vi "ALTS-2015 Auto Mode.vi"() -> ()   [LabVIEW 2013]
doc: "Copyright © 2005, Soliton Technologies.\nAll rights reserved."
uses:
  Controls/ALTS-2015 Station Details.ctl
  Controls/ALTS-2015 Status Ring Indicator.ctl
  Controls/ALTS-2015 Robot Actions.ctl
  SLL DAQ Engine/Software/Source Code/Sub VIs/DAQ Engine/Controls/SLL DE List of Digital Inputs.ctl
  Controls/ALTS-2015 Auto Main Screen States.ctl
  Sub VIs/OPC Engine/Controls/ALTS-2015 OPC Global Elements.ctl
  Sub VIs/OPC Engine/Controls/ALTS-2015 OPC Global Options.ctl
  Controls/ALTS-2015 Data Cluster.ctl
  Controls/ALTS-2015 Station Cluster.ctl
  Controls/ALTS-2015 INI Configuration Cluster.ctl
  Controls/ALTS-2015 Unload Task Data.ctl
  Controls/ALTS-2015 Status Message Options.ctl
  Controls/ALTS-2015 LV2GBL WorkOrder&SN Info Options.ctl
  Controls/ALTS-2015 LV2GBL Options.ctl
  Controls/ALTS-2015 WorkOrder&SN Cluster.ctl
  Controls/ALTS-2015 Control Reference LV2 Options.ctl
  Controls/ALTS-2015 Control Reference.ctl
  SLL DAQ Engine/Software/Source Code/Sub VIs/DAQ Engine/Controls/SLL DE DI Global Options.ctl
  Controls/ALTS-2015 LV2GBL Restart Options.ctl
  Controls/ALTS-2015 LV2 Options.ctl
  <vilib>/Utility/error.llb/DialogType.ctl
  SLL DAQ Engine/Software/Source Code/Sub VIs/DAQ Engine/Controls/SLL DE DO Global Options.ctl
  Controls/ALTS-2015 Auto Program States.ctl
  Sub VIs/Robot Controller Queue/ALTS-2015 Robot Cotroller Options.ctl
  SLL DAQ Engine/Software/Source Code/Sub VIs/DAQ Engine/Controls/SLL DE DAQ Global Options.ctl
  SLL DAQ Engine/Software/Source Code/Sub VIs/DAQ Engine/Controls/SLL DE DAQ Global Elements.ctl
  Controls/ALTS-2015 DO Start Stop Options.ctl
  Controls/ALTS-2015 LV2GBL Station Info Options.ctl
  Controls/ALTS-2015 Ring Indicator Enum.ctl
  Controls/ALTS-2015 Digital Output Options.ctl
  Controls/ALTS-2015 DB Driver Options.ctl
  Controls/ALTS-2015 Robot Tasks.ctl
  Controls/ALTS-2015 Serial Details.ctl
  Controls/ALTS-2015 Serial DB Details.ctl
  Controls/ALTS-2015 Serial Task Handler FGV-Command.ctl
  Controls/ALTS-2015 Write DB Write Result Driver Cases.ctl
  Controls/ALTS-2015 Bundle Cluster for DB Result Options.ctl
  Controls/ALTS-2015 write DB Result cases.ctl
  Globals/ALTS-2015 Global Variables.vi
  Sub VIs/OPC Engine/Globals/ALTS-2015 OPC Engine Globals.vi
panel:
  in  "Error Message":string
  out "User :":string caption="Date :"
  in  "Login/Logoff":bool
  in  "Restart":bool
  out "Status":string
  out "Error Occured":bool
  in  "Open Manual Screen":bool
  in  "List of Digital Inputs":T1
  out "Time :":string
  out "Date :":string
  in  "DI Status":bool[](array[boolean])
  out "Last Scanned Serial Number":string caption="Status"
  out "Station Cluster 4":T2={"Station Number"="", "Work Order Number"="", "Sensor Name"="", "Pressure (PSI)"="", "Flow (SCCM)"="", "Test Time "="", "Test Result"="", "Serial Number"="", "Station Status"=0, "SW assigned UUT"=FALSE, "Rerun Count"=0, "Test Type"=0, "Load Decision"=0, "Robot Action"=enum."No Action"}
  out "Station Cluster 3":T2={"Station Number"="", "Work Order Number"="", "Sensor Name"="", "Pressure (PSI)"="", "Flow (SCCM)"="", "Test Time "="", "Test Result"="", "Serial Number"="", "Station Status"=0, "SW assigned UUT"=FALSE, "Rerun Count"=0, "Test Type"=0, "Load Decision"=0, "Robot Action"=enum."No Action"}
  out "Station Cluster 2":T2={"Station Number"="", "Work Order Number"="", "Sensor Name"="", "Pressure (PSI)"="", "Flow (SCCM)"="", "Test Time "="", "Test Result"="", "Serial Number"="", "Station Status"=0, "SW assigned UUT"=FALSE, "Rerun Count"=0, "Test Type"=0, "Load Decision"=0, "Robot Action"=enum."No Action"}
  out "Station Cluster 1":T2={"Station Number"="", "Work Order Number"="", "Sensor Name"="", "Pressure (PSI)"="", "Flow (SCCM)"="", "Test Time "="", "Test Result"="", "Serial Number"="", "Station Status"=0, "SW assigned UUT"=FALSE, "Rerun Count"=0, "Test Type"=0, "Load Decision"=0, "Robot Action"=enum."No Action"}
  in  "Exit":bool
  out "error out":errorcluster
  in  "error in":errorcluster
  # "Air Leak Test System (Auto)"
  # "V 3.0.2"
  # "Dont delete these Controls. Its Property Nodes are used"
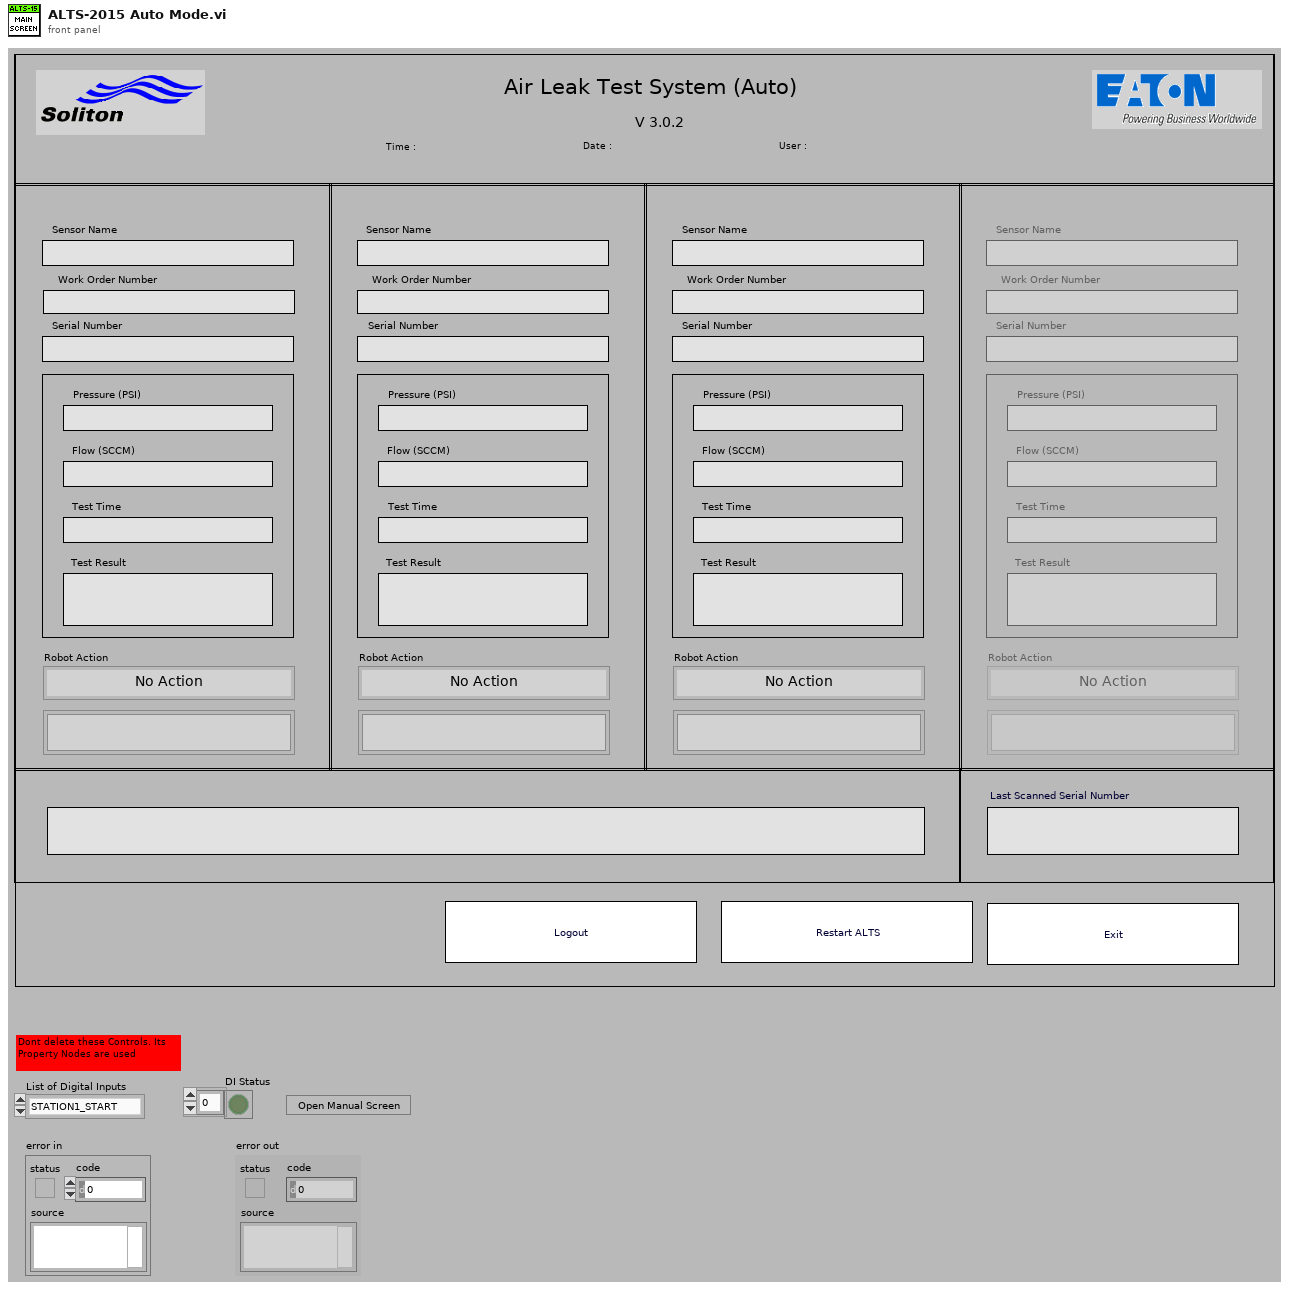
[diagram p1: front panel]
types:
  T1 = typedef "SLL DE List of Digital Inputs.ctl" = enum16{"STATION1_START", "STATION1_STOP", "STATION1_CLAMPED", "STATION1_TC_PASS", "STATION1_TC_FAIL", "STATION1_TTA", "STATION1_TTB", "STATION2_START", "STATION2_STOP", "STATION2_CLAMPED", "STATION2_TC_PASS", "STATION2_TC_FAIL", "STATION2_TTA", "STATION2_TTB", "STATION3_START", "STATION3_STOP", "STATION3_CLAMPED", "STATION3_TC_PASS", "STATION3_TC_FAIL", "STATION3_TTA", "STATION3_TTB", "STATION4_START", "STATION4_STOP", "STATION4_CLAMPED", "STATION4_TC_PASS", "STATION4_TC_FAIL", "STATION4_TTA", "STATION4_TTB"}
  T2 = typedef "ALTS-2015 Station Details.ctl" = cluster{"Station Number":string, "Work Order Number":string, "Sensor Name":string, "Pressure (PSI)":string, "Flow (SCCM)":string, "Test Time ":string, "Test Result":string, "Serial Number":string, "Station Status":T3, "SW assigned UUT":bool, "Rerun Count":i32, "Test Type":i32, "Load Decision":i32, "Robot Action":T4}
  T3 = typedef "ALTS-2015 Status Ring Indicator.ctl" = u16
  T4 = typedef "ALTS-2015 Robot Actions.ctl" = enum16{"Loading...", "Unloading...", "Reruning...", "No Action"}
  T5 = enum16{"Init", "Set - DB Loop", "Set - Robot Loop", "Get"}
  T6 = typedef "ALTS-2015 Auto Main Screen States.ctl" = enum16{">Initialize", ">Poll", ">Error", ">Exit", ">Restart", ">Authentication", ">Check Robot Requests", ">Scan Serial No", "<-------DI /OPC Actions------->", ">Check DI Status", ">Start the Test", ">Restore station after Stop", ">Stop the Test", ">UUT Clamped", ">UUT Unclamped", ">Read Test Data Result - Pass", ">Read Test Data Result - Fail", ">Update Rerun on Fail", ">Update Station Info", "<--------Enqueue Robot Task-------->", ">Enqueue New Serial Task", ">Enqueue Invalid Serial Task", ">Enqueue Rerun Task", ">Enqueu Unload Task"}
  T7 = enum16{"Init", "Set Task Pass", "Set Task Failure", "Set Task Status", "Get"}
  T8 = typedef "ALTS-2015 Control Reference.ctl" = cluster{"User :":refnum<vi>, "Station Cluster 1":refnum<vi>, "Station Cluster 2":refnum<vi>, "Station Cluster 3":refnum<vi>, "Station Cluster 4":refnum<vi>, "Error Message":refnum<vi>, "Login/Logoff":refnum<vi>}
  T9 = typedef "ALTS-2015 Control Reference LV2 Options.ctl" = enum16{"Set", "Get"}
  T10 = enum32{"invalid app kind", "Development System", "Run Time System", "Student Edition", "Embedded LabVIEW", "Evaluation", "Custom"}
  T11 = typedef "ALTS-2015 WorkOrder&SN Cluster.ctl" = cluster{"Work Order Number":string}
  T12 = typedef "ALTS-2015 LV2GBL Options.ctl" = enum16{"Read all", "Write all"}
  T13 = typedef "ALTS-2015 LV2GBL WorkOrder&SN Info Options.ctl" = enum16{"Init", "Read all", "Write Work Order"}
  T14 = typedef "ALTS-2015 Status Message Options.ctl" = enum16{"Initializing...", "Enter User Login...", "Valid Serial Number...", "Invalid Serial Number...", "Start Tag Received...", "Stop Tag Received...", "UUT Clamped...", "UUT not Clamped...", "Test Running...", "Test Complete...", "Task is assigned to robot...", "Robot is working on the task...", "Robot is ready for next task...", "Writing Result to DB...", "Idle...", "Exiting..."}
  T15 = typedef "SLL DE DI Global Options.ctl" = enum16{"Init", "Write Line", "Write Array", "Read Line", "Read Array", "Read Full Status", "Write Full Status"}
  T16 = typedef "ALTS-2015 LV2GBL Restart Options.ctl" = enum16{"Get All Data", "Set Restart Notifier Ref", "Store Authentication Data"}
  T17 = enum32{"Invalid", "Standard", "Closed", "Hidden", "Minimized", "Maximized"}
  T18 = typedef "ALTS-2015 LV2 Options.ctl" = enum16{"Get", "Set"}
  T19 = typedef "SLL DE DAQ Global Elements.ctl" = enum16{"AI Error", "AO Error", "DI Error", "DO Error", "AI Restart", "DI Restart", "AI Running", "AO Running", "DI Running", "DO Running", "DAQ Exit?"}
  T20 = typedef "SLL DE DAQ Global Options.ctl" = enum16{"Init", "Write 1", "Read 1", "Write Array", "Read Array", "Clear"}
  T21 = typedef "ALTS-2015 Robot Cotroller Options.ctl" = enum16{"Init", "Enqueue State", "Enqueue State in Opposite End", "Dequeue State", "Exit"}
  T22 = typedef "ALTS-2015 Auto Program States.ctl" = enum16{"<------ Robot Handler States ------>", "Wait for Robot Availability", "Check Last Task by Robot", "Wait & Read Task from Queue", "Write New Task Details to Robot", "Write Task Available for Robot", "Check Robot for Unavailbilty", "Write Task Unavailable for Robot", "<------------ Other ------------>", "Error", "Exit"}
  T23 = typedef "ALTS-2015 Station Cluster.ctl" = enum16{"Station 1", "Station 2", "Station 3", "Station 4"}
  T24 = cluster{"Test Status":string, "Station Name":T23}
  T25 = typedef "SLL DE DO Global Options.ctl" = enum16{"Init", "Write Line", "Write Array", "Write Full Status", "Read Line", "Read Array", "Read Full Status", "Restart DO", "Send to Safe Mode", "Stop DO"}
  T26 = typedef "ALTS-2015 DO Start Stop Options.ctl" = enum16{"Start Test", "Stop Test"}
  T27 = typedef "ALTS-2015 Digital Output Options.ctl" = enum16{"Idle", "Test Running", "Pass", "Fail"}
  T28 = typedef "ALTS-2015 Ring Indicator Enum.ctl" = enum16{"Idle", "Test Running", "Unit Clamped", "Unit not Clamped", "Pass", "Fail"}
  T29 = typedef "ALTS-2015 LV2GBL Station Info Options.ctl" = enum16{"Init", "Read", "Read All", "Write Sensor ID", "Write  Work Order", "Write Serial Number", "Write Test Data", "Write Station Status", "Write Station Occupancy", "Write Station Test Type", "Write Rerun", "Write Load Decision", "Write Robot Action", "Clear All", "Clear Test Result"}
  T30 = typedef "ALTS-2015 Unload Task Data.ctl" = cluster{"Station to Unload":T23, "Test Result":bool}
  T31 = typedef "ALTS-2015 Serial Task Handler FGV-Command.ctl" = enum16{"Set Replace/Insert Falg", "Get Status", "Reset Flag", "Reset S Data"}
  T32 = typedef "ALTS-2015 Robot Tasks.ctl" = enum16{"Load", "Unload", "Rerun", "Invalid Serial"}
  T33 = typedef "ALTS-2015 DB Driver Options.ctl" = enum16{"Init", "Read DB", "Close"}
  T34 = typedef "ALTS-2015 Data Cluster.ctl" = cluster{"Serial No":string, "DI Change Status":bool[], "Station Selected":T23[], "Station to Start Stop Test":T23, "INI Info":T35, "Stations to Rerun":T23[], "Unload Task":T30[], "Dev. System?":bool, "Manual Restart?":bool}
  T35 = typedef "ALTS-2015 INI Configuration Cluster.ctl" = cluster{"Application":cluster{"Rerun Count":i32, "Workorder No":string, "PLC Scanner":bool, "Time Delay to Restart(mins)":dbl}, "Station Details":cluster{"Sensor Name 1":string, "Sensor Name 2":string, "Sensor Name 3":string, "Sensor Name 4":string, "Station1 Enable":bool, "Station2 Enable":bool, "Station3 Enable":bool, "Station4 Enable":bool}, "Database":cluster{"Database Connection Link":path, "Result Procedure":string, "User":string, "Password":string, "Prompt":bool, "Station 1 LT Result DB DSN Path":path, "Station 2 LT Result DB DSN Path":path, "Station 3 LT Result DB DSN Path":path, "Station 4 LT Result DB DSN Path":path, "AirLeakTestResult Procedure":string, "Serial Details Procedure":string}, "Simulation":cluster{"Simulate DAQ Hardware":bool, "Simulate Result DB Write":bool, "Simulate Scanner":bool, "Simulate OPC":bool, "Simulate Serial Details DB":bool, "Simulate Result DB":bool, "Simulate Scanner DB Path":path, "Simulate Serial Details DB Path":path, "Simulate Result DB Path":path}, "Barcode Scanner1":cluster{"Scanner IP":string, "Scanner Port":u16, "#Bytes to Read":i32, "Timeout_ms":i32}, "Barcode Scanner2":cluster{"Enabled?":bool, "Scanner IP":string, "Scanner Port":u16, "#Bytes to Read":i32}}
  T36 = typedef "DialogType.ctl" = u16
  T37 = cluster{"Station Cluster":T23, "Last Test Result":bool}
  T38 = typedef "ALTS-2015 Serial Details.ctl" = cluster{"Robot Task":T32, "Serial No":string, "New Serial?":bool, "Station # Unload":T23, "Last Test Result":bool, "Rerun?":bool, "Station # Rerun":T23, "Invalid Serial?":bool, "Serial Details":T39}
  T39 = typedef "ALTS-2015 Serial DB Details.ctl" = cluster{"Adapter Plate Size":i32, "Air Leak Test Type ":i32, "Displacement Size":i32, "Flange Size":i32, "Height":i32, "Load Decision":i32, "Cart Insert":i32}
  T40 = typedef "ALTS-2015 OPC Global Elements.ctl" = enum16{"OPC - R Error", "OPC - W Error", "OPC - R Restart", "OPC - W Restart", "OPC - R Running", "OPC - W Running"}
  T41 = typedef "ALTS-2015 OPC Global Options.ctl" = enum16{"Init", "Write 1", "Read 1", "Write Array", "Read Array", "Clear"}
  T42 = typedef "ALTS-2015 write DB Result cases.ctl" = enum16{"Enter All Data", "Enter WO & SN"}
  T43 = typedef "ALTS-2015 Bundle Cluster for DB Result Options.ctl" = enum16{"Write", "Read"}
  T44 = typedef "ALTS-2015 Write DB Write Result Driver Cases.ctl" = enum16{"Init", "Write Result", "Close"}
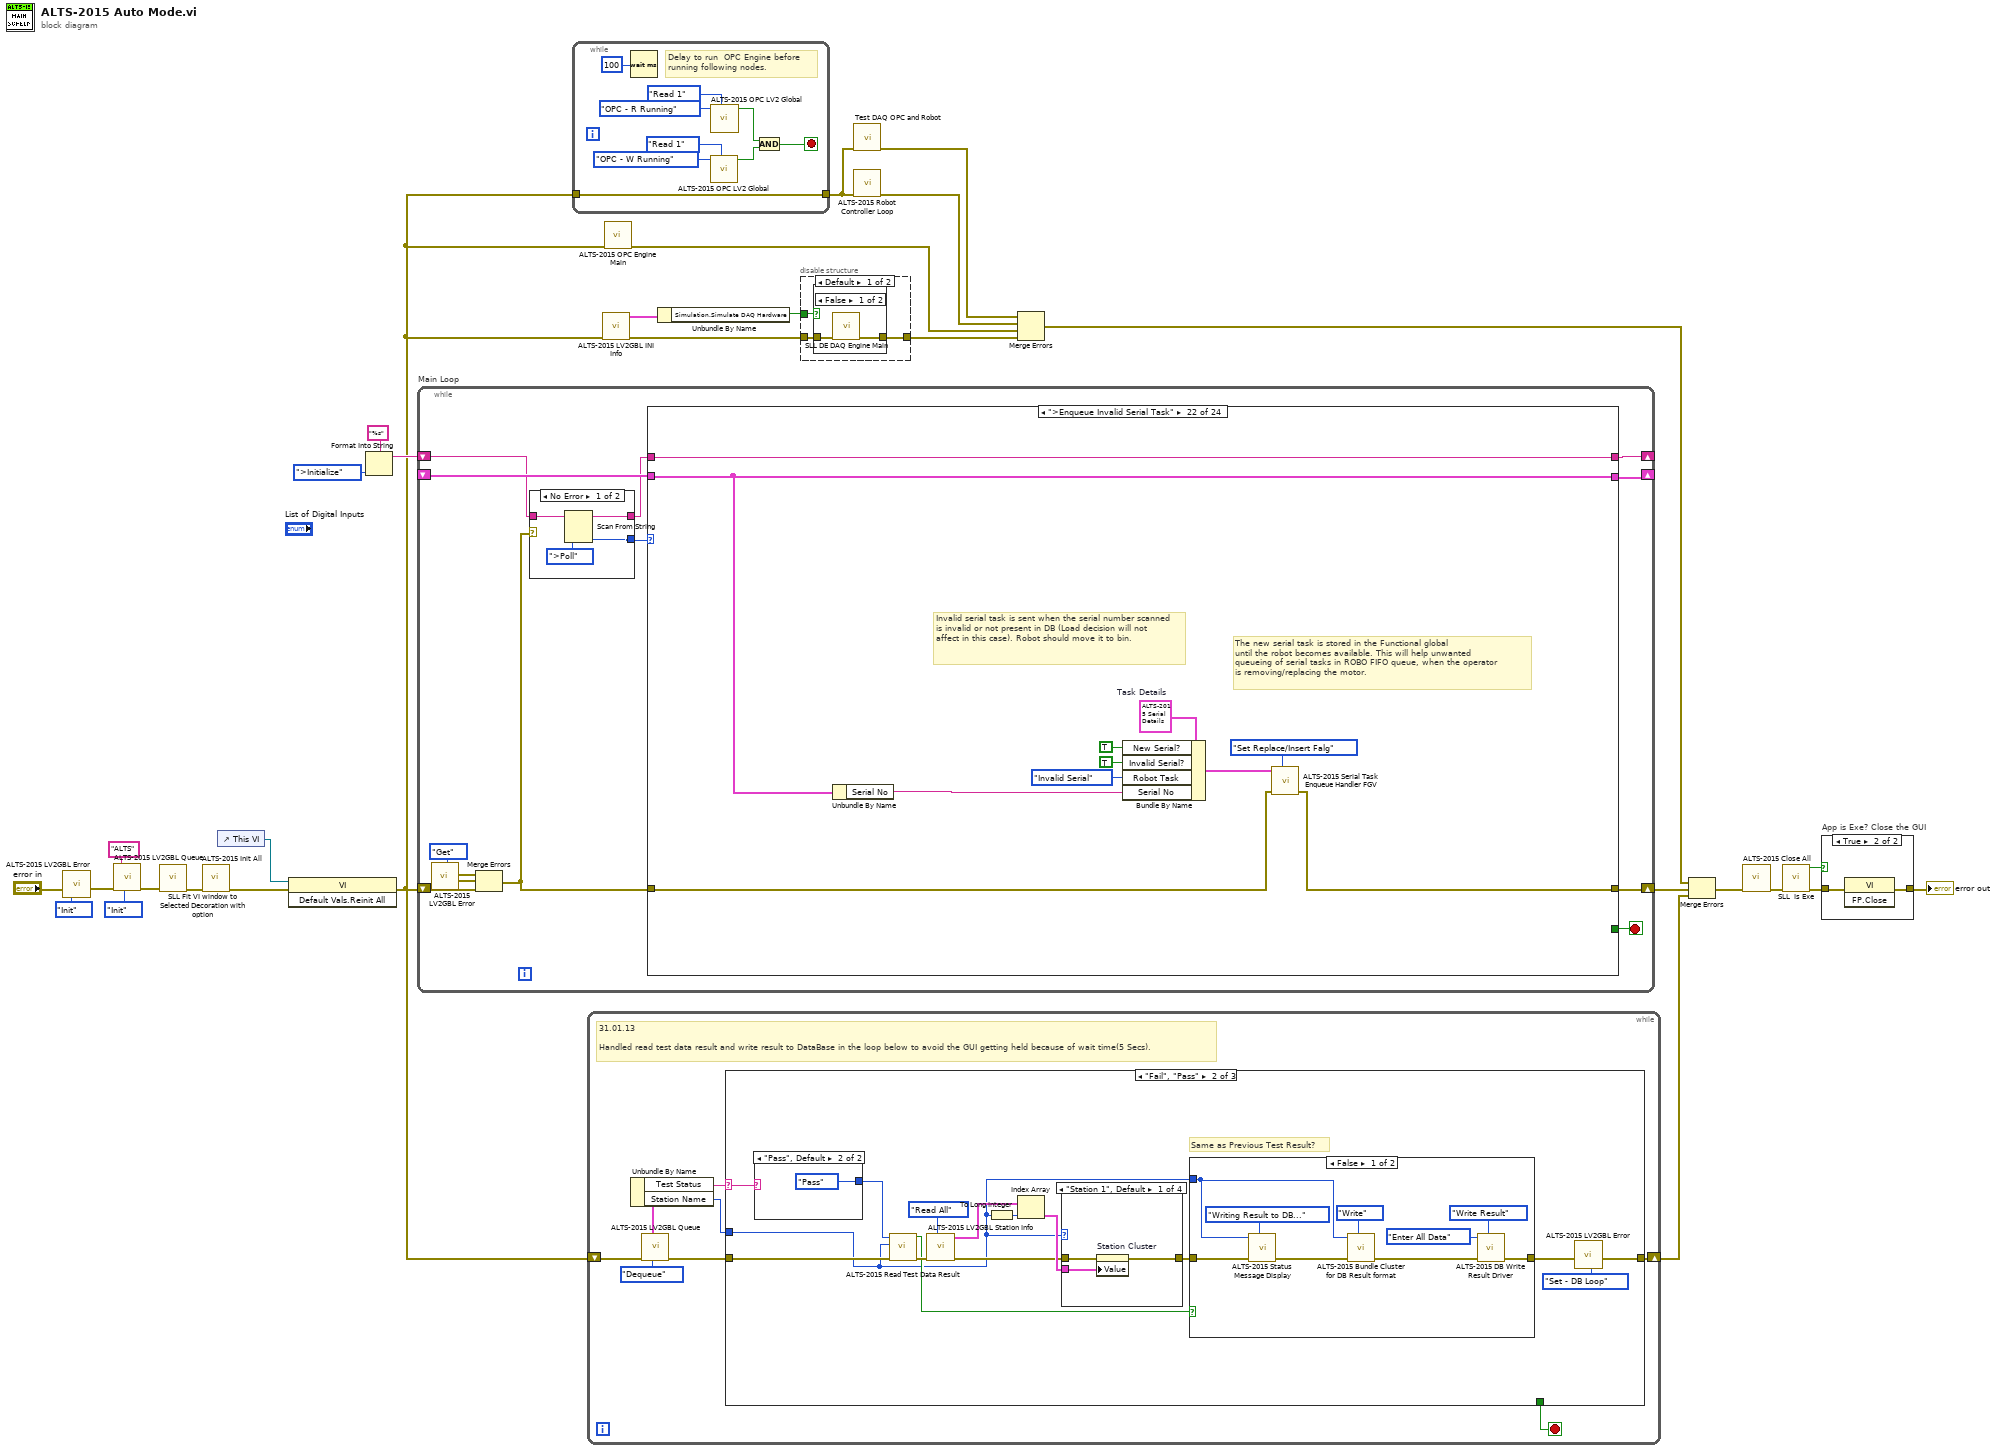
[diagram p0: block diagram]
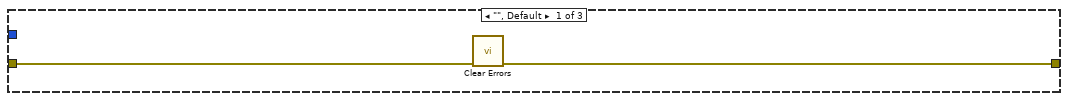
[diagram p5: hidden frame]
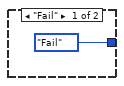
[diagram p6: hidden frame]
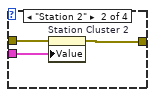
[diagram p8: hidden frame]
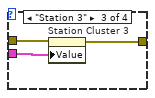
[diagram p9: hidden frame]
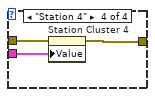
[diagram p10: hidden frame]
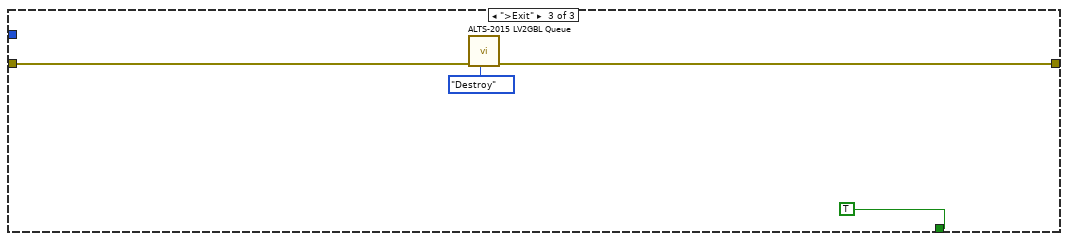
[diagram p11: hidden frame]
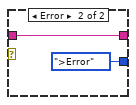
[diagram p12: hidden frame]
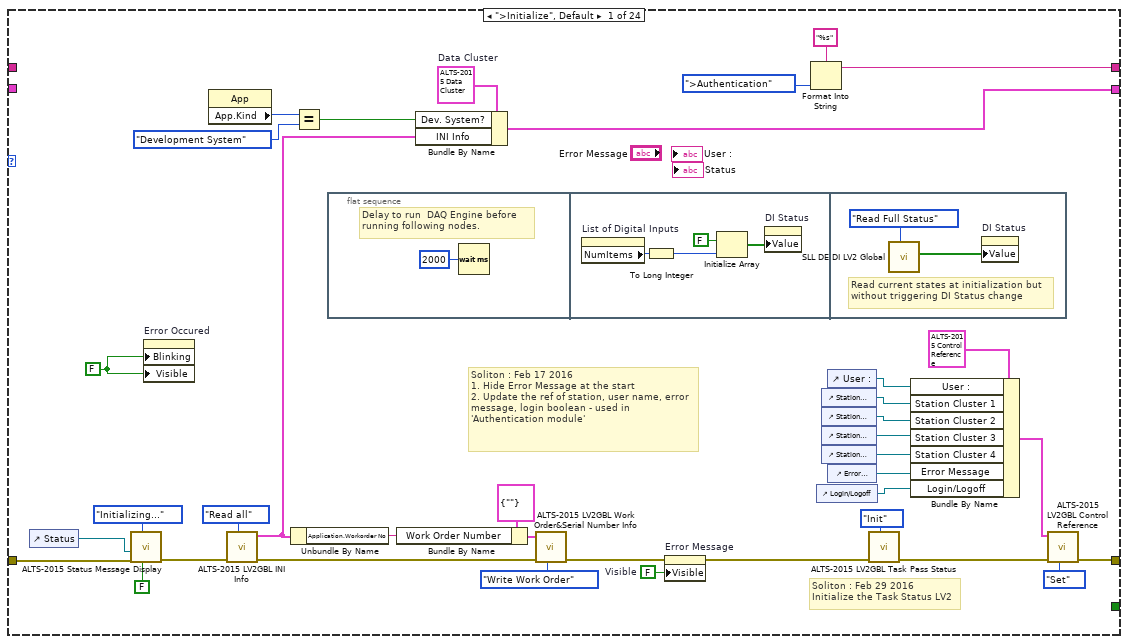
[diagram p13: hidden frame]
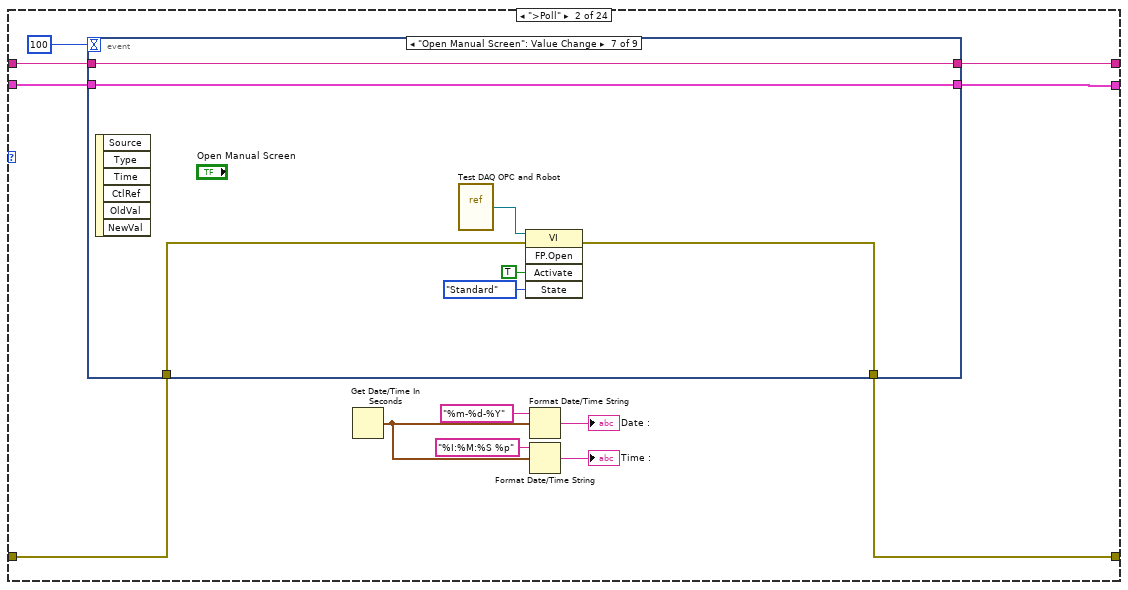
[diagram p14: hidden frame]
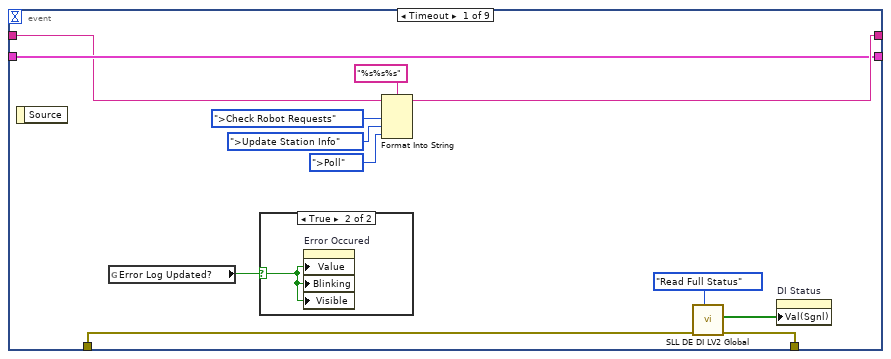
[diagram p15: hidden frame]
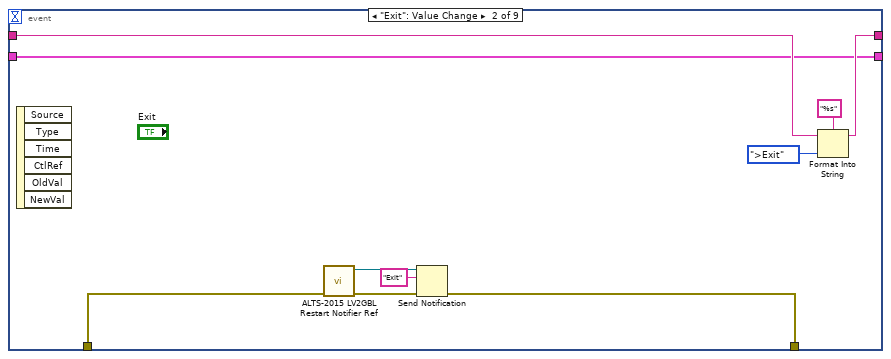
[diagram p17: hidden frame]
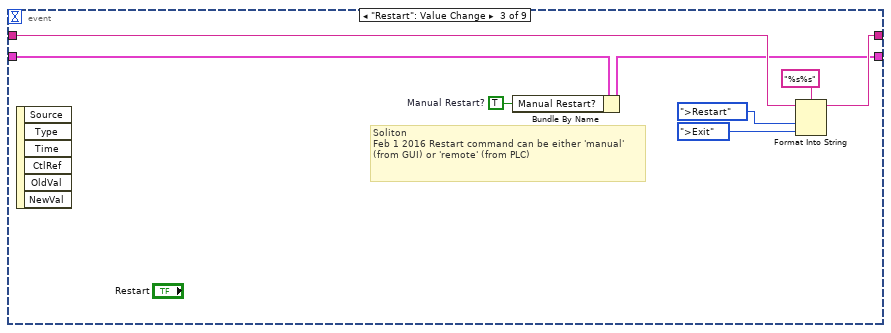
[diagram p18: hidden frame]
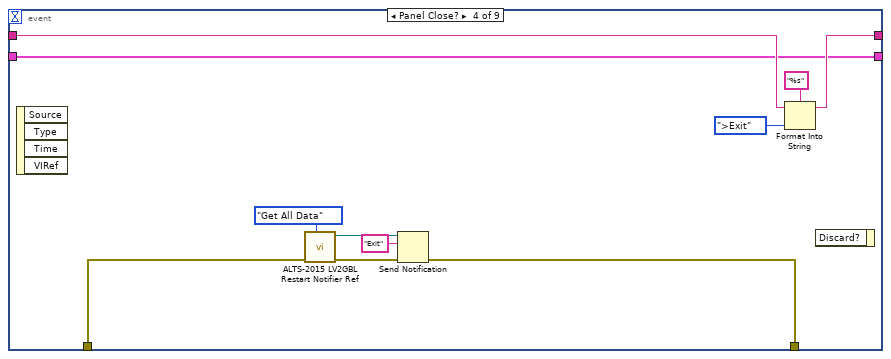
[diagram p19: hidden frame]
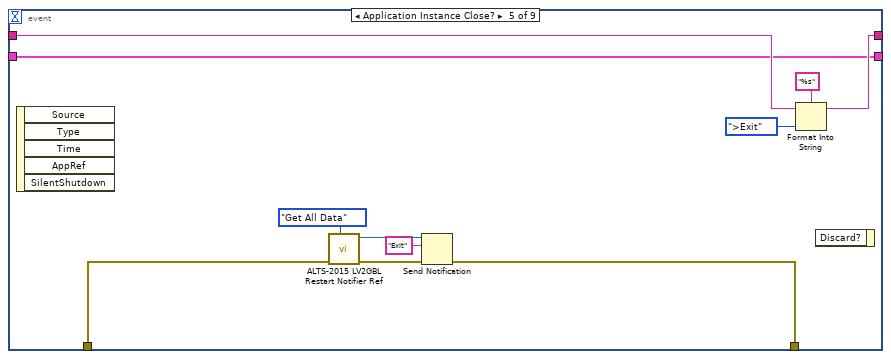
[diagram p20: hidden frame]
diagram:
  n1 = call "ALTS-2015 LV2GBL Error.vi"("error in - DB Loop"="error in", "Operation"=T5."Init") -> ("error out  - DB Loop"=w27:errorcluster)  [unwired: 8 in, 1 out]
  n2 = call "ALTS-2015 LV2GBL Queue.vi"("Enum"=enum16{"Init", "Enqueue", "Dequeue", "Destroy"}."Init", "error in (no error)"=w27, "Queue name"="ALTS") -> ("error out"=w23:errorcluster)  [unwired: 7 in, 1 out]
  n3 = call "SLL Fit VI window to Selected Decoration with option.vi"("error in (no error)"=w23) -> ("error out"=w22:errorcluster)  [unwired: 9 in, 1 out]
  n4 = call "ALTS-2015 Init All.vi"("error in"=w22) -> ("error out"=w13:errorcluster)  [unwired: 10 in]
  n5 = control-ref of="This VI"() -> (w4:refnum<vi>)
  n6 = invoke class="VI" method="Default Vals.Reinit All"(reference=w4, error in=w13) -> (error out=w5:errorcluster)  [unwired: 1 in, 2 out]
  n7 = Format Into String(format string="%s", ALTS-2015_Auto_Main_Screen_States.">Initialize") -> (resulting string=w17:string)  [unwired: 2 in, 1 out]
  n8 = while "Main Loop" {
    shift-right: [w42] -> _
    shift-left: w17 -> [w36]
    shift-right: [w40] -> w18
    shift-left: w5 -> [w31]
    shift-right: [w39] -> _
    shift-left: _ -> [w38]
    stop <- w37 stop-if-true
    n9 = call "ALTS-2015 LV2GBL Error.vi"("Operation"=T5."Get") -> ("error out  - DB Loop"=w32:errorcluster, "error out  - Robot Loop"=w34:errorcluster)  [unwired: 9 in]
    n10 = Merge Errors(w34, w32, w31) -> (w30:errorcluster)
    n11 = case shown="No Error" w30 {
      tunnel: [w45 ALTS-2015_Auto_Main_Screen_States.">Error"] -> w41
      tunnel: w36 -> [w44 w48]
      tunnel: [w43 w48] -> w35
      frame No Error {
        n12 = Scan From String(input string=w44, default 1=ALTS-2015_Auto_Main_Screen_States.">Poll") -> (remaining string=w43:string, output 1=w45:T6)  [unwired: 3 in, 2 out]
      }
      frame Error {
      }
    }
    n13 = case shown="\">Enqueue Invalid Serial Task\"" w41 {
      tunnel: [w81 w103 w239 w270 w283 w299 w305 w310 w318 w327 w349 w358 w389 w398 w410 w427 w446 w468 w501 w511 w518 w536 w537 w554] -> w42
      tunnel: w35 -> [_ w102 w239 w270 w283 w299 w305 w311 w312 w328 w349 w358 w389 w398 w410 w428 w446 w467 w501 w511 w518 w536 w538 w555]
      tunnel: [w64 w93 w230 w247 w281 w301 w304 w306 w314 w324 w348 w352 w367 w390 w405 w433 w447 w461 w497 w510 w522 w531 w544 w558] -> w40
      tunnel: w30 -> [w79 w104 w238 w249 w280 w300 w304 w307 w315 w323 w345 w354 w371 w391 w406 w421 w443 w462 w498 w510 w524 w535 w545 w560]
      tunnel: [w72 w99 w237 w269 w275 w302 w303 w308 w316 w321 w347 w350 w372 w392 w403 w431 w445 w458 w496 w509 w521 w528 w541 w556] -> w39
      tunnel: w38 -> [_ w100 w237 w269 w275 w302 w303 w309 w317 w322 w347 w351 w373 w393 w404 w432 w448 w460 w496 w509 w521 w528 w543 w559]
      tunnel: [_ _ _ TRUE ("Exit") _ _ _ _ _ _ _ _ _ _ _ _ _ _ _ _ _ _ _ _] -> w37
      frame ">Initialize", Default {
        w53 = FALSE  # Visible
        w65 = FALSE ("Blinking")
        w85 = T34 {"Serial No"="", "DI Change Status"=[], "Station Selected"=[], "Station to Start Stop Test"=enum."Station 1", "INI Info"={"Application"={"Rerun Count"=0, "Workorder No"="", "PLC Scanner"=FALSE, "Time Delay to Restart(mins)"=0.0}, "Station Details"={"Sensor Name 1"="", "Sensor Name 2"="", "Sensor Name 3"="", "Sensor Name 4"="", "Station1 Enable"=FALSE, "Station2 Enable"=FALSE, "Station3 Enable"=FALSE, "Station4 Enable"=FALSE}, "Database"={"Database Connection Link"=path "", "Result Procedure"="", "User"="", "Password"="", "Prompt"=FALSE, "Station 1 LT Result DB DSN Path"=path "", "Station 2 LT Result DB DSN Path"=path "", "Station 3 LT Result DB DSN Path"=path "", "Station 4 LT Result DB DSN Path"=path "", "AirLeakTestResult Procedure"="", "Serial Details Procedure"=""}, "Simulation"={"Simulate DAQ Hardware"=FALSE, "Simulate Result DB Write"=FALSE, "Simulate Scanner"=FALSE, "Simulate OPC"=FALSE, "Simulate Serial Details DB"=FALSE, "Simulate Result DB"=FALSE, "Simulate Scanner DB Path"=path "", "Simulate Serial Details DB Path"=path "", "Simulate Result DB Path"=path ""}, "Barcode Scanner1"={"Scanner IP"="", "Scanner Port"=0, "#Bytes to Read"=0, "Timeout_ms"=0}, "Barcode Scanner2"={"Enabled?"=FALSE, "Scanner IP"="", "Scanner Port"=0, "#Bytes to Read"=0}}, "Stations to Rerun"=[], "Unload Task"=[], "Dev. System?"=FALSE, "Manual Restart?"=FALSE}  # Data Cluster
        # "Soliton : Feb 29 2016\nInitialize the Task Status LV2"
        # "Soliton : Feb 17 2016\n1. Hide Error Message at the start\n2. Update the ref of station, user name, error message, login boolean - used in 'Authentication module'"
        n14 = control-ref of="Status"() -> (w69:refnum<vi>)
        n15 = call "ALTS-2015 Status Message Display.vi"("Station Message?"=FALSE, "Status Message Options"=ALTS-2015_Status_Message_Options."Initializing...", "error in (no error)"=w79, "Status Message"=w69) -> ("error out"=w70:errorcluster)  [unwired: 6 in, 1 out]
        n16 = property on="Error Occured" class="Bool (strict)"("Blinking"=w65, "Visible"=w65) -> ()  [unwired: 2 in, 2 out]
        n17 = property class="App"() -> ("App.Kind"=w67:T10)  [unwired: 2 in, 2 out]
        n18 = call "ALTS-2015 LV2GBL INI Info.vi"("Options"=ALTS-2015_LV2GBL_Options."Read all", "error in"=w70) -> ("error out"=w73:errorcluster, "Configuration Cluster Out"=w71:T35)  [unwired: 8 in]
        n19 = Unbundle By Name(w71) -> ("Application.Workorder No"=w74:string)
        n20 = Equal?(x=w67, y=T10."Development System" ("Application:Kind")) -> (x = y?=w66:bool)
        n21 = flat-sequence {
          frame #0 {
            # "Delay to run  DAQ Engine before\nrunning following nodes."
            n22 = Wait (ms)(milliseconds to wait=u32 2000) -> ()  [unwired: 1 out]
          }
          frame #1 {
            n23 = property on="List of Digital Inputs" class="Enum (strict)"() -> ("NumItems"=w88:u32)  [unwired: 2 in, 2 out]
            n24 = To Long Integer(number=w88) -> (32bit integer=w87:i32)
            n25 = Initialize Array(FALSE ("Key Focus"), w87) -> (w89:bool[])
            n26 = property on="DI Status" class="Arr (strict)"("Value"=w89) -> ()  [unwired: 2 in, 2 out]
          }
          frame #2 {
            # "Read current states at initialization but\nwithout triggering DI Status change"
            n27 = call "SLL DE DI LV2 Global.vi"("Option"=SLL_DE_DI_Global_Options."Read Full Status") -> ("Digital Array Status"=w91:bool[])  [unwired: 7 in, 3 out]
            n28 = property on="DI Status" class="Arr (strict)"("Value"=w91) -> ()  [unwired: 2 in, 2 out]
          }
        }
        n29 = Bundle By Name(cluster=T11 {"Work Order Number"=""} ("Work Order&SN Cluster In"), "Work Order Number"=w74) -> (w75:T11)
        n30 = Bundle By Name(cluster=w85, "Dev. System?"=w66, "INI Info"=w71) -> (w72:T34)
        n31 = call "ALTS-2015 LV2GBL Work Order&Serial Number Info.vi"("Options"=ALTS-2015_LV2GBL_WorkOrder&SN_Info_Options."Write Work Order", "error in"=w73, "Work Order&SN Cluster In"=w75) -> ("error out"=w52:errorcluster)  [unwired: 7 in, 1 out]
        n32 = property on="Error Message" class="Str"(error in=w52, "Visible"=w53) -> (error out=w51:errorcluster)  [unwired: 1 in, 1 out]
        n33 = Format Into String(format string="%s", ALTS-2015_Auto_Main_Screen_States.">Authentication") -> (resulting string=w81:string)  [unwired: 2 in, 1 out]
        n34 = control-ref of="Login/Logoff"() -> (w54:refnum<vi>)
        n35 = control-ref of="Station Cluster 1"() -> (w60:refnum<vi>)
        n36 = control-ref of="Station Cluster 2"() -> (w59:refnum<vi>)
        n37 = control-ref of="Station Cluster 3"() -> (w58:refnum<vi>)
        n38 = control-ref of="Station Cluster 4"() -> (w57:refnum<vi>)
        n39 = control-ref of="User :"() -> (w61:refnum<vi>)
        n40 = control-ref of="Error Message"() -> (w56:refnum<vi>)
        n41 = call "ALTS-2015 LV2GBL Task Pass Status.vi"("Options"=T7."Init", "error in"=w51) -> ("error out"=w50:errorcluster)  [unwired: 7 in, 2 out]
        n42 = Bundle By Name(cluster=T8 {"User :"=refnum, "Station Cluster 1"=refnum, "Station Cluster 2"=refnum, "Station Cluster 3"=refnum, "Station Cluster 4"=refnum, "Error Message"=refnum, "Login/Logoff"=refnum} ("Control Reference_In"), "User :"=w61, "Station Cluster 1"=w60, "Station Cluster 2"=w59, "Station Cluster 3"=w58, "Station Cluster 4"=w57, "Error Message"=w56, "Login/Logoff"=w54) -> (w55:T8)
        n43 = call "ALTS-2015 LV2GBL Control Reference.vi"("LV2 Options"=ALTS-2015_Control_Reference_LV2_Options."Set", "error in"=w50, "Control Reference_In"=w55) -> ("error out"=w64:errorcluster)  [unwired: 7 in, 1 out]
      }
      frame ">Poll" {
        n44 = event shown="[6] \"Open Manual Screen\": Value Change" {
          selector: _ -> [_ _ _ _ _ _ _ _ _]
          dyn-events: _ -> [_ _ _ _ _ _ _ _ _]
          timeout: 100 -> [_ _ _ _ _ _ _ _ _]
          tunnel: [w114 w126 w133 w144 w155 w165 w177 w187 w201] -> w103
          tunnel: w102 -> [w112 w124 w134 w143 w154 w160 w177 w187 w202]
          tunnel: w100 -> [w113 w123 w130 w142 w153 w161 w178 w186 w204]
          tunnel: [w113 w123 w129 w142 w153 w162 w178 w186 w204] -> w99
          tunnel: w104 -> [w109 w119 _ w137 w148 w159 w180 w188 w199]
          tunnel: [w111 w121 _ w139 w147 w158 w179 w191 w198] -> w93
          event Timeout {
            n45 = event-data() -> ()  [unwired: 1 in, 1 out]
            n46 = global read "ALTS-2015 Global Variables.vi" "Error Log Updated?"() -> (w110:bool)
            n47 = case shown="True" w110 {
              selector: w110 -> [_ w117]
              frame False {
              }
              frame True {
                n48 = property on="Error Occured" class="Bool (strict)"("Value"=w117, "Blinking"=w117, "Visible"=w117) -> ()  [unwired: 2 in, 2 out]
              }
            }
            n49 = Format Into String(format string="%s%s%s", initial string=w112, ALTS-2015_Auto_Main_Screen_States.">Check Robot Requests", ALTS-2015_Auto_Main_Screen_States.">Update Station Info" ("input 2"), ALTS-2015_Auto_Main_Screen_States.">Poll" ("input 2")) -> (resulting string=w114:string)  [unwired: 1 in, 1 out]
            n50 = call "SLL DE DI LV2 Global.vi"("Option"=SLL_DE_DI_Global_Options."Read Full Status", "error in (no error)"=w109) -> ("error out"=w111:errorcluster, "Digital Array Status"=w115:bool[])  [unwired: 6 in, 2 out]
            n51 = property on="DI Status" class="Arr (strict)"("Val(Sgnl)"=w115) -> ()  [unwired: 2 in, 2 out]
          }
          event "Exit": Value Change {
            n52 = event-data() -> ()  [unwired: 1 in, 6 out]
            n53 = call "ALTS-2015 LV2GBL Restart Notifier Ref.vi"("Error In"=w119) -> ("Error Out"=w120:errorcluster, "Restart Notifier Out"=w118:refnum<notifier>)  [unwired: 8 in, 1 out]
            n54 = Send Notification(notification="Exit", notifier=w118, error in (no error)=w120) -> (error out=w121:errorcluster)  [unwired: 1 out]
            n55 = Format Into String(format string="%s", initial string=w124, ALTS-2015_Auto_Main_Screen_States.">Exit") -> (resulting string=w126:string)  [unwired: 1 in, 1 out]
          }
          event "Restart": Value Change {
            w128 = TRUE  # Manual Restart?
            # "Soliton\nFeb 1 2016 Restart command can be either 'manual' (from GUI) or 'remote' (from PLC)"
            n56 = event-data() -> ()  [unwired: 1 in, 6 out]
            n57 = Bundle By Name(cluster=w130, "Manual Restart?"=w128) -> (w129:T34)
            n58 = Format Into String(format string="%s%s", initial string=w134, ALTS-2015_Auto_Main_Screen_States.">Restart" ("input 1"), ALTS-2015_Auto_Main_Screen_States.">Exit") -> (resulting string=w133:string)  [unwired: 1 in, 1 out]
          }
          event Panel Close? {
            n59 = event-data() -> ()  [unwired: 1 in, 4 out]
            n60 = call "ALTS-2015 LV2GBL Restart Notifier Ref.vi"("Options"=ALTS-2015_LV2GBL_Restart_Options."Get All Data", "Error In"=w137) -> ("Error Out"=w138:errorcluster, "Restart Notifier Out"=w140:refnum<notifier>)  [unwired: 7 in, 1 out]
            n61 = Send Notification(notification="Exit", notifier=w140, error in (no error)=w138) -> (error out=w139:errorcluster)  [unwired: 1 out]
            n62 = Format Into String(format string="%s", initial string=w143, ALTS-2015_Auto_Main_Screen_States.">Exit") -> (resulting string=w144:string)  [unwired: 1 in, 1 out]
            n63 = event-data() -> ()  [unwired: 2 in, 1 out]
          }
          event Application Instance Close? {
            n64 = event-data() -> ()  [unwired: 1 in, 5 out]
            n65 = call "ALTS-2015 LV2GBL Restart Notifier Ref.vi"("Options"=ALTS-2015_LV2GBL_Restart_Options."Get All Data", "Error In"=w148) -> ("Error Out"=w150:errorcluster, "Restart Notifier Out"=w151:refnum<notifier>)  [unwired: 7 in, 1 out]
            n66 = Send Notification(notification="Exit", notifier=w151, error in (no error)=w150) -> (error out=w147:errorcluster)  [unwired: 1 out]
            n67 = Format Into String(format string="%s", initial string=w154, ALTS-2015_Auto_Main_Screen_States.">Exit") -> (resulting string=w155:string)  [unwired: 1 in, 1 out]
            n68 = event-data() -> ()  [unwired: 2 in, 1 out]
          }
          event "DI Status": Value Change {
            n69 = event-data() -> ("OldVal"=w164:bool[], "NewVal"=w163:bool[])  [unwired: 1 in, 4 out]
            n70 = call "ALTS-2015 LV2GBL DI status Info.vi"("Options"=ALTS-2015_LV2GBL_Options."Write all", "error in"=w159, "DI Status"=w163) -> ("error out"=w158:errorcluster)  [unwired: 7 in, 1 out]
            n71 = Not Equal?(x=w164, y=w163) -> (x != y?=w168:bool[])
            n72 = Or Array Elements(Boolean array=w168) -> (logical OR=w167:bool)
            n73 = case "DI Change?" shown="True" w167 {
              tunnel: [w169 w176] -> w165
              tunnel: [w170 w173] -> w162
              tunnel: w168 -> [_ w175]
              tunnel: w161 -> [w170 w174]
              tunnel: w160 -> [w169 w171]
              frame False {
              }
              frame True {
                n74 = Bundle By Name(cluster=w174, "DI Change Status"=w175) -> (w173:T34)
                n75 = Format Into String(initial string=w171, ALTS-2015_Auto_Main_Screen_States.">Check DI Status") -> (resulting string=w176:string)  [unwired: 2 in, 1 out]
              }
            }
          }
          event "Open Manual Screen": Value Change {
            n76 = event-data() -> ()  [unwired: 1 in, 6 out]
            n77 = vi-ref "Test DAQ OPC and Robot.vi"() -> (w183:refnum<vi>)
            n78 = invoke class="VI" method="FP.Open"(reference=w183, error in=w180, "Activate"=TRUE ("Activate?"), "State"=T17."Standard") -> (error out=w179:errorcluster)  [unwired: 1 in, 4 out]
          }
          event "Error Occured": Mouse Down {
            w185 = FALSE ("Error Occured")
            n79 = event-data() -> ()  [unwired: 1 in, 8 out]
            n80 = call "ALTS-2015 File and folder info.vi"("error in (no error)"=w188) -> ("Error Log file Path Out"=w189:path, "error out"=w190:errorcluster)  [unwired: 9 in, 8 out]
            n81 = Strip Path(path=w189) -> (stripped path=w192:path, name=w196:string)
            n82 = Concatenate Strings("notepad.exe \"" ("command line"), w196, "\"" ("string")) -> (w195:string)
            n83 = call <vilib>:"System Exec.vi"("wait until completion? (T)"=FALSE, "error in (no error)"=w190, "working directory"=w192, "command line"=w195) -> ("error out"=w193:errorcluster)  [unwired: 4 in, 3 out]
            n84 = call <vilib>:"Clear Errors.vi"("error in (no error)"=w193) -> ("error out"=w191:errorcluster)  [unwired: 6 in]
            n85 = property on="Error Occured" class="Bool (strict)"("Blinking"=w185, "Visible"=w185) -> ()  [unwired: 2 in, 2 out]
            n86 = global write "ALTS-2015 Global Variables.vi" "Error Log Updated?"(w185) -> ()
            "Error Occured" <- w185
          }
          event "Login/Logoff": Value Change {
            # "Soliton : Feb 17 2016\nHandle login/logout button press"
            n87 = event-data() -> ()  [unwired: 1 in, 6 out]
            n88 = property on="Login/Logoff" class="Bool"(error in=w199) -> (error out=w200:errorcluster, "BoolText.Text"=w203:string)  [unwired: 1 in, 1 out]
            n89 = case "Boolean Text - Login?" shown="\"Login\"" w203 {
              tunnel: w202 -> [w220 w222 w226]
              tunnel: [w220 w222 w225] -> w201
              tunnel: w200 -> [w209 w221 w224]
              tunnel: [w205 w221 w223] -> w198
              frame "Logout" {
                w208 = TRUE  # Visible
                n90 = property on="Login/Logoff" class="Bool"(error in=w209, "TipStrip"="Press to Login" ("Tip Strip"), "BoolText.Text"="Login" ("Boolean Text.Text")) -> (error out=w210:errorcluster)  [unwired: 1 in, 1 out]
                n91 = property on="User :" class="Str"(error in=w210, "Value"="" ("User :")) -> (error out=w212:errorcluster)  [unwired: 1 in, 1 out]
                n92 = call "ALTS-2015 LV2GBL Restart Notifier Ref.vi"("Options"=ALTS-2015_LV2GBL_Restart_Options."Store Authentication Data", "Error In"=w212, "Authenticated User Name"="") -> ("Error Out"=w211:errorcluster)  [unwired: 6 in, 2 out]
                n93 = call "ALTS-2015 LV2GBL Login Status.vi"("Options"=ALTS-2015_LV2_Options."Set", "error in (no error)"=w211, "Login Status?"=FALSE) -> ("error out"=w206:errorcluster)  [unwired: 7 in, 1 out]
                n94 = property on="Error Message" class="Str"(error in=w206, "Visible"=w208, "Blinking"=w208, "Value"="Login to Test" ("Error Message")) -> (error out=w205:errorcluster)  [unwired: 1 in, 1 out]
              }
              frame Default {
              }
              frame "Login" {
                # "When boolean status is 'login', enqueue 'Authentication' state"
                n95 = Format Into String(format string="%s", initial string=w226, error in=w224, ALTS-2015_Auto_Main_Screen_States.">Authentication") -> (resulting string=w225:string, error out=w223:errorcluster)
              }
            }
          }
        }
        n96 = Get Date/Time In Seconds() -> (seconds since 1Jan1904=w96:timestamp)
        n97 = Format Date/Time String(time format string (%c)="%m-%d-%Y", seconds (now)=w96) -> (date/time string=→"Date :":string)  [unwired: 1 in]
        n98 = Format Date/Time String(time format string (%c)="%I:%M:%S %p", seconds (now)=w96) -> (date/time string=→"Time :":string)  [unwired: 1 in]
      }
      frame ">Error" {
        n99 = Unbundle By Name(w237) -> ("Dev. System?"=w236:bool)
        n100 = case shown="True" w236 {
          tunnel: w238 -> [w240 w243]
          tunnel: [w240 w242] -> w231
          frame False {
            # "No error popping in runtime mode"
          }
          frame True {
            w241 = T36 2 items=["no dialog", "OK message", "continue or stop message", "OK message + warnings", "continue/stop + warnings"] ("type of dialog (OK msg:1)")
            n101 = call <vilib>:"Simple Error Handler.vi"("type of dialog (OK msg:1)"=w241, "error in (no error)"=w243) -> ("error out"=w242:errorcluster)  [unwired: 3 in, 4 out]
          }
        }
        n102 = call "ALTS-2015 Get_ErrorString.vi"("Incoming Error"=w231) -> ("error out"=w235:errorcluster, "Message"=w234:string)  [unwired: 9 in]
        n103 = Concatenate Strings("Error occured at \"Auto Mode .vi\"\n" ("string"), w234) -> (w233:string)
        n104 = call "ALTS-2015 Write Status Log.vi"("error in (no error)"=w235, "Status Input"=w233) -> ("error out"=w230:errorcluster)  [unwired: 9 in]
        n105 = call "ALTS-2015 LV2GBL Error.vi"("Operation"=T5."Init") -> ()  [unwired: 9 in, 2 out]
      }
      frame ">Exit" {
        # "Soliton : Feb 17 2016\n Hide Error Message at the exit"
        # "Before Exit send safe values to the DO"
        n106 = call "ALTS-2015 Status Message Display.vi"("Station Message?"=FALSE, "Status Message Options"=ALTS-2015_Status_Message_Options."Exiting...", "error in (no error)"=w249) -> ("error out"=w246:errorcluster)  [unwired: 7 in, 1 out]
        n107 = property on="Error Message" class="Str"(error in=w246, "Visible"=FALSE) -> (error out=w245:errorcluster)  [unwired: 1 in, 1 out]
        n108 = disable-structure shown="Default" {
          disable-tunnel: w245 -> [w272 w273]
          disable-tunnel: [w271 w273] -> w248
          frame condition #0 (active) {
            n109 = call "ALTS-2015 Set Test Type 1.vi"("error in"=w272) -> ("error out"=w271:errorcluster)  [unwired: 10 in]
          }
          frame condition #1 {
          }
        }
        n110 = call "SLL DE DO LV2 Global.vi"("DO Option"=SLL_DE_DO_Global_Options."Send to Safe Mode", "Error In"=w248) -> ("error out"=w254:errorcluster)  [unwired: 6 in, 3 out]
        n111 = global write "ALTS-2015 OPC Engine Globals.vi" "OPC Exit?"(TRUE ("OPC Exit?")) -> ()
        n112 = global write "ALTS-2015 Global Variables.vi" "Exit Troubleshooter VI"(TRUE ("Exit Troubleshooter VI")) -> ()
        n113 = call "ALTS-2015 Copy Text To Clipboard.vi"("Text to copy to clipboard"="") -> ()  [unwired: 1 out]
        n114 = call "SLL DE DAQ LV2 Global.vi"("Option"=SLL_DE_DAQ_Global_Options."Write 1", "error in (no error)"=w254, "Status In"=TRUE, "Element"=SLL_DE_DAQ_Global_Elements."DAQ Exit?") -> ("error out"=w253:errorcluster)  [unwired: 5 in, 2 out]
        n115 = call "ALTS-2015 Robot State Controller.vi"("Option"=ALTS-2015_Robot_Cotroller_Options."Enqueue State", "error in"=w253, "Enqueue State"=ALTS-2015_Auto_Program_States."Exit") -> ("error out"=w259:errorcluster)  [unwired: 7 in, 1 out]
        n116 = Bundle By Name(cluster=T24 {"Test Status"="", "Station Name"=enum."Station 1"} ("Enqueue Element"), "Test Status"=">Exit") -> (w263:T24)
        n117 = call "ALTS-2015 LV2GBL Queue.vi"("Enum"=enum16{"Init", "Enqueue", "Dequeue", "Destroy"}."Enqueue", "error in (no error)"=w259, "Enqueue Element"=w263) -> ("error out"=w247:errorcluster)  [unwired: 7 in, 1 out]
      }
      frame ">Restart" {
        n118 = Unbundle By Name(w275) -> ("Manual Restart?"=w274:bool)
        n119 = case "'Restart' button clicked manually?" shown="False" w274 {
          tunnel: [w285 w290] -> w279
          tunnel: w280 -> [w285 w288]
          frame True {
            n120 = One Button Dialog(message="Please reset the robot and make sure that it is in the home position and all stations have been cleared!!!!") -> ()  [unwired: 1 in, 1 out]
          }
          frame False {
            n121 = call "ALTS-2015 LV2GBL INI Info.vi"("error in"=w288) -> ("error out"=w287:errorcluster, "Configuration Cluster Out"=w289:T35)  [unwired: 9 in]
            n122 = Unbundle By Name(w289) -> ("Application.Time Delay to Restart(mins)"=w286:dbl)
            n123 = call "ALTS-2015 Show Remaining Time .vi"("error in (no error)"=w287, "Time Delay to Restart (Mins)"=w286) -> ("error out"=w290:errorcluster)  [unwired: 9 in]
          }
        }
        n124 = call "ALTS-2015 LV2GBL Restart Notifier Ref.vi"("Options"=ALTS-2015_LV2GBL_Restart_Options."Get All Data", "Error In"=w279) -> ("Error Out"=w278:errorcluster, "Restart Notifier Out"=w277:refnum<notifier>)  [unwired: 7 in, 1 out]
        n125 = Send Notification(notification="LaunchMainVI", notifier=w277, error in (no error)=w278) -> (error out=w281:errorcluster)  [unwired: 1 out]
      }
      frame ">Authentication" {
        w291 = TRUE  # Auto Dispose Reference
        w292 = FALSE  # Wait until done
        w294 = FALSE  # Show FP?
        # "Soliton : Feb 17 2016\n'Login/Logout' button press shouldnot affect normal normal flow of the test; hence launched dynamically"
        n126 = call <vilib>:"Clear Errors.vi"("error in (no error)"=w300) -> ("error out"=w298:errorcluster)  [unwired: 6 in]
        n127 = Current VI's Path() -> (path=w297:path)
        n128 = Build Path(base path=w297, name or relative path="..\\Sub VIs\\ALTS-2015 Authentication Module.vi") -> (appended path=w295:path)
        n129 = call "ALTS-2015 Load VI Dynamically v1.0.vi"("Auto Dispose Reference"=w291, "Show FP?"=w294, "Wait until done"=w292, "error in"=w298, "VI Path"=w295) -> ("error out"=w293:errorcluster)  [unwired: 6 in]
        n130 = Merge Errors(w293, w300) -> (w301:errorcluster)
      }
      frame "<-------DI /OPC Actions------->" {
      }
      frame ">Check Robot Requests" {
        n131 = call "ALTS-2015 Check Robot Requests.vi"("error in (no error)"=w307, "Data Cluster in"=w309, "Cases to go In"=w311) -> ("error out"=w306:errorcluster, "Data Cluster out"=w308:T34, "Cases to go Out"=w310:string)  [unwired: 6 in]
      }
      frame ">Check DI Status" {
        n132 = Unbundle By Name(w317) -> ("DI Change Status"=w313:bool[])
        n133 = call "ALTS-2015 Decide Cases to go.vi"("error in"=w315, "DI Change Status"=w313, "Cases to go In"=w312) -> ("error out"=w314:errorcluster, "Station Selected"=w319:T23[], "Cases to go Out"=w318:string)  [unwired: 6 in]
        n134 = Bundle By Name(cluster=w317, "Station Selected"=w319) -> (w316:T34)
      }
      frame ">Scan Serial No" {
        n135 = call "ALTS-2015-Read Serial Number.vi"("error in (no error)"=w323) -> ("error out"=w325:errorcluster, "Valid Serial Number?"=w326:bool, "Serial No"=w320:string)  [unwired: 8 in]
        "Last Scanned Serial Number" <- w320
        n136 = case "Valid S.No?" shown="False" w326 {
          tunnel: [w334 w340] -> w327
          tunnel: w328 -> [w335 w339]
          tunnel: w325 -> [w329 w336]
          tunnel: [w329 w336] -> w324
          frame False {
            # "S.No is valid but does not\nexist in DB"
            n137 = Format Into String(format string="%s", initial string=w335, ALTS-2015_Auto_Main_Screen_States.">Enqueue Invalid Serial Task") -> (resulting string=w334:string)  [unwired: 1 in, 1 out]
            n138 = call "ALTS-2015 Status Message Display.vi"("Station Message?"=FALSE, "Status Message Options"=ALTS-2015_Status_Message_Options."Invalid Serial Number...") -> ()  [unwired: 8 in, 2 out]
          }
          frame True {
            n139 = Format Into String(format string="%s", initial string=w339, ALTS-2015_Auto_Main_Screen_States.">Enqueue New Serial Task") -> (resulting string=w340:string)  [unwired: 1 in, 1 out]
            n140 = call "ALTS-2015 Status Message Display.vi"("Station Message?"=FALSE, "Status Message Options"=ALTS-2015_Status_Message_Options."Valid Serial Number...") -> ()  [unwired: 8 in, 2 out]
          }
        }
        n141 = Bundle By Name(cluster=w322, "Serial No"=w320) -> (w321:T34)
      }
      frame ">Start the Test" {
        n142 = Unbundle By Name(w347) -> ("Station to Start Stop Test"=w343:T23)
        n143 = call "ALTS-2015 Status Message Display.vi"("Status Message Options"=ALTS-2015_Status_Message_Options."Start Tag Received...", "error in (no error)"=w345, "Station Enum"=w343) -> ("error out"=w344:errorcluster)  [unwired: 7 in, 1 out]
        n144 = call "ALTS-2015 Start Test.vi"("error in (no error)"=w344, "Station Cluster"=w343) -> ("error out"=w348:errorcluster)  [unwired: 9 in]
      }
      frame ">Stop the Test" {
        n145 = disable-structure shown="Disabled" {
          disable-tunnel: [w363 w366] -> w356
          disable-tunnel: w351 -> [w360 w365]
          disable-tunnel: [w359 w365] -> w350
          frame Disabled {
            n146 = Unbundle By Name(w360) -> ("Station Selected"=w361:T23[])
            n147 = Delete From Array "Delete From Array"(array=w361, index=0) -> (deleted portion=w363:T23, array with subset deleted=w362:T23[])  [unwired: 1 in]
            n148 = Bundle By Name(cluster=w360, "Station Selected"=w362) -> (w359:T34)
          }
          frame Enabled {
            n149 = Unbundle By Name(w365) -> ("Station to Start Stop Test"=w366:T23)
          }
        }
        n150 = call "ALTS-2015 Status Message Display.vi"("Status Message Options"=ALTS-2015_Status_Message_Options."Stop Tag Received...", "error in (no error)"=w354, "Station Enum"=w356) -> ("error out"=w353:errorcluster)  [unwired: 7 in, 1 out]
        n151 = call "ALTS-2015 Update Start Stop DO.vi"("DO Options"=ALTS-2015_DO_Start_Stop_Options."Stop Test", "error in"=w353, "Station Cluster"=w356) -> ("error out"=w352:errorcluster)  [unwired: 8 in]
      }
      frame ">Restore station after Stop" {
        n152 = Unbundle By Name(w373) -> ("Station Selected"=w374:T23[])
        n153 = Delete From Array "Delete From Array"(array=w374, index=0) -> (deleted portion=w387:T23, array with subset deleted=w375:T23[])  [unwired: 1 in]
        n154 = call "ALTS-2015 Check for Clamp Status .vi"("error in (no error)"=w371, "Station Cluster"=w387) -> ("error out"=w370:errorcluster, "Clamp?"=w385:bool)  [unwired: 8 in]
        n155 = call "ALTS-2015 LV2GBL Station Info.vi"("Options"=ALTS-2015_LV2GBL_Station_Info_Options."Read", "error in"=w370) -> ("error out"=w369:errorcluster, "Station Details"=w381:T2)  [unwired: 7 in, 1 out]
        n156 = Select(t=ALTS-2015_Ring_Indicator_Enum."Unit Clamped" ("Ring Indicator Options"), s=w385, f=ALTS-2015_Ring_Indicator_Enum."Idle" ("Ring Indicator Options")) -> (s? t:f=w382:T28)
        n157 = Type Cast(type=T3 0 ("Station Status"), x=w382) -> (*(type *) &x=w380:T3)
        n158 = Bundle By Name(cluster=w381, "Station Status"=w380) -> (w378:T2)
        n159 = Bundle By Name(cluster=w373, "Station Selected"=w375) -> (w372:T34)
        n160 = call "ALTS-2015 LV2GBL Station Info.vi"("Options"=ALTS-2015_LV2GBL_Station_Info_Options."Write Station Status", "error in"=w369, "Station"=w378, "Station Cluster"=w387) -> ("error out"=w368:errorcluster)  [unwired: 5 in, 2 out]
        n161 = call "ALTS-2015 Update Status Light Indicator.vi"("DO Options"=ALTS-2015_Digital_Output_Options."Idle", "error in"=w368, "Station Cluster"=w387) -> ("error out"=w367:errorcluster)  [unwired: 8 in]
      }
      frame ">UUT Clamped" {
        n162 = Unbundle By Name(w393) -> ("Station Selected"=w394:T23[])
        n163 = Delete From Array "Delete From Array"(array=w394, index=0) -> (deleted portion=w396:T23, array with subset deleted=w395:T23[])  [unwired: 1 in]
        n164 = call "ALTS-2015 UUT clamped.vi"("error in"=w391, "Station Cluster"=w396) -> ("error out"=w390:errorcluster)  [unwired: 9 in]
        n165 = Bundle By Name(cluster=w393, "Station Selected"=w395) -> (w392:T34)
      }
      frame ">UUT Unclamped" {
        # "Unclamped?"
        n166 = Unbundle By Name(w404) -> ("Station Selected"=w407:T23[])
        n167 = Delete From Array "Delete From Array"(array=w407, index=0) -> (deleted portion=w401:T23, array with subset deleted=w408:T23[])  [unwired: 1 in]
        n168 = call "ALTS-2015 Check for Clamp Status .vi"("error in (no error)"=w406, "Station Cluster"=w401) -> ("error out"=w402:errorcluster, "Clamp?"=w400:bool)  [unwired: 8 in]
        n169 = Not(x=w400) -> (.not. x?=w399:bool)
        n170 = case "Unclamped?" shown="True" w399 {
          tunnel: w401 -> [_ w415]
          tunnel: w402 -> [w411 w417]
          tunnel: [w411 w416] -> w405
          frame False {
          }
          frame True {
            # "Clears Test Data\non Rerun"
            n171 = call "ALTS-2015 Update Clamp Status.vi"("error in"=w417, "Station Cluster"=w415) -> ("error out"=w413:errorcluster)  [unwired: 9 in]
            n172 = call "ALTS-2015 LV2GBL Station Info.vi"("Options"=ALTS-2015_LV2GBL_Station_Info_Options."Write Test Data", "error in"=w413) -> ("error out"=w412:errorcluster)  [unwired: 7 in, 2 out]
            n173 = call "ALTS-2015 Update Status Light Indicator.vi"("DO Options"=ALTS-2015_Digital_Output_Options."Idle", "error in"=w412, "Station Cluster"=w415) -> ("error out"=w416:errorcluster)  [unwired: 8 in]
          }
        }
        n174 = Bundle By Name(cluster=w404, "Station Selected"=w408) -> (w403:T34)
      }
      frame ">Read Test Data Result - Pass" {
        w424 = TRUE  # Last Test Result
        n175 = Unbundle By Name(w432) -> ("Unload Task"=w426:T30[], "Station Selected"=w434:T23[])
        n176 = Delete From Array "Delete From Array"(array=w434, index=0) -> (deleted portion=w419:T23, array with subset deleted=w436:T23[])  [unwired: 1 in]
        n177 = call "ALTS-2015 Status Message Display.vi"("Status Message Options"=ALTS-2015_Status_Message_Options."Test Complete...", "error in (no error)"=w421, "Station Enum"=w419) -> ("error out"=w420:errorcluster)  [unwired: 7 in, 1 out]
        n178 = Bundle("Station Cluster"=w419, "Last Test Result"=w424) -> (w423:T37)  [unwired: 1 in]
        n179 = Insert Into Array(array=w426, new element=w423) -> (w425:T30[])  [unwired: 1 in]
        n180 = Bundle By Name(cluster=T24 {"Test Status"="", "Station Name"=enum."Station 1"} ("Enqueue Element"), "Test Status"="Pass", "Station Name"=w419) -> (w438:T24)
        n181 = Bundle By Name(cluster=w432, "Unload Task"=w425, "Station Selected"=w436) -> (w431:T34)
        n182 = call "ALTS-2015 LV2GBL Queue.vi"("Enum"=enum16{"Init", "Enqueue", "Dequeue", "Destroy"}."Enqueue", "error in (no error)"=w420, "Enqueue Element"=w438) -> ("error out"=w433:errorcluster)  [unwired: 7 in, 1 out]
        n183 = Format Into String(format string="%s", initial string=w428, ALTS-2015_Auto_Main_Screen_States.">Enqueu Unload Task") -> (resulting string=w427:string)  [unwired: 1 in, 1 out]
      }
      frame ">Read Test Data Result - Fail" {
        n184 = Unbundle By Name(w448) -> ("Station Selected"=w449:T23[])
        n185 = Delete From Array "Delete From Array"(array=w449, index=0) -> (deleted portion=w441:T23, array with subset deleted=w452:T23[])  [unwired: 1 in]
        n186 = call "ALTS-2015 Status Message Display.vi"("Status Message Options"=ALTS-2015_Status_Message_Options."Test Complete...", "error in (no error)"=w443, "Station Enum"=w441) -> ("error out"=w442:errorcluster)  [unwired: 7 in, 1 out]
        n187 = Bundle By Name(cluster=T24 {"Test Status"="", "Station Name"=enum."Station 1"} ("Enqueue Element"), "Test Status"="Fail", "Station Name"=w441) -> (w454:T24)
        n188 = Bundle By Name(cluster=w448, "Station Selected"=w452) -> (w445:T34)
        n189 = call "ALTS-2015 LV2GBL Queue.vi"("Enum"=enum16{"Init", "Enqueue", "Dequeue", "Destroy"}."Enqueue", "error in (no error)"=w442, "Enqueue Element"=w454) -> ("error out"=w447:errorcluster)  [unwired: 7 in, 1 out]
      }
      frame ">Update Rerun on Fail" {
        n190 = Unbundle By Name(w460) -> ("Stations to Rerun"=w465:T23[], "Unload Task"=w464:T30[], "INI Info.Application.Rerun Count"=w463:i32, "Station Selected"=w459:T23[])
        n191 = Delete From Array "Delete From Array"(array=w459, index=0) -> (deleted portion=w471:T23, array with subset deleted=w476:T23[])  [unwired: 1 in]
        n192 = call "ALTS-2015 LV2GBL Station Info.vi"("Options"=ALTS-2015_LV2GBL_Station_Info_Options."Read", "error in"=w462, "Station Cluster"=w471) -> ("error out"=w461:errorcluster, "Station Details"=w473:T2)  [unwired: 6 in, 1 out]
        n193 = Unbundle By Name(w473) -> ("Rerun Count"=w470:i32)
        n194 = Greater?(x=w463, y=w470) -> (0:w472:bool)
        n195 = case "Rerun Count not reached?" shown="True" w472 {
          tunnel: w471 -> [w481 w494]
          tunnel: w470 -> [w486 _]
          tunnel: w464 -> [w479 w492]
          tunnel: w465 -> [w477 w488]
          tunnel: [ALTS-2015_Auto_Main_Screen_States.">Enqueue Rerun Task" ALTS-2015_Auto_Main_Screen_States.">Enqueu Unload Task"] -> w466
          tunnel: [w478 w488] -> w457
          tunnel: [w479 w489] -> w456
          frame True {
            n196 = Increment(x=w486) -> (x+1=w482:i32)
            n197 = Insert Into Array(array=w477, new element=w481) -> (w478:T23[])  [unwired: 1 in]
            n198 = Bundle By Name(cluster=T2 {"Station Number"="", "Work Order Number"="", "Sensor Name"="", "Pressure (PSI)"="", "Flow (SCCM)"="", "Test Time "="", "Test Result"="", "Serial Number"="", "Station Status"=0, "SW assigned UUT"=FALSE, "Rerun Count"=0, "Test Type"=0, "Load Decision"=0, "Robot Action"=enum."Loading..."} ("Station"), "Rerun Count"=w482) -> (w484:T2)
            n199 = call "ALTS-2015 LV2GBL Station Info.vi"("Options"=ALTS-2015_LV2GBL_Station_Info_Options."Write Rerun", "Station"=w484, "Station Cluster"=w481) -> ()  [unwired: 6 in, 3 out]
          }
          frame False {
            w493 = FALSE  # Last Test Result
            n200 = Bundle By Name(cluster=T30 {"Station to Unload"=enum."Station 1", "Test Result"=FALSE}, "Station to Unload"=w494, "Test Result"=w493) -> (w491:T30)
            n201 = Insert Into Array(array=w492, new element=w491) -> (w489:T30[])  [unwired: 1 in]
          }
        }
        n202 = Format Into String(format string="%s", initial string=w467, w466) -> (resulting string=w468:string)  [unwired: 1 in, 1 out]
        n203 = Bundle By Name(cluster=w460, "Stations to Rerun"=w457, "Unload Task"=w456, "Station Selected"=w476) -> (w458:T34)
      }
      frame ">Update Station Info" {
        n204 = call "ALTS-2015 LV2GBL Station Info.vi"("Options"=ALTS-2015_LV2GBL_Station_Info_Options."Read All", "error in"=w498) -> ("error out"=w497:errorcluster, "Station Info Array"=w500:T2[])  [unwired: 7 in, 1 out]
        n205 = for {
          N: 4 -> [_]
          tunnel: w500 -> [w503]
          i -> [w502]
          n206 = Index Array(array=w503, index=w502) -> (element=w504:T2)
          n207 = case shown="0, Default" w502 {
            tunnel: w504 -> [w505 w506 w507 w508]
            frame 0, Default {
              "Station Cluster 1" <- w505
            }
            frame 1 {
              "Station Cluster 2" <- w506
            }
            frame 2 {
              "Station Cluster 3" <- w507
            }
            frame 3 {
              "Station Cluster 4" <- w508
            }
          }
        }
      }
      frame "<--------Enqueue Robot Task-------->" {
      }
      frame ">Enqueue New Serial Task" {
        w517 = T38 {"Robot Task"=enum."Load", "Serial No"="", "New Serial?"=FALSE, "Station # Unload"=enum."Station 1", "Last Test Result"=FALSE, "Rerun?"=FALSE, "Station # Rerun"=enum."Station 1", "Invalid Serial?"=FALSE, "Serial Details"={"Adapter Plate Size"=0, "Air Leak Test Type "=0, "Displacement Size"=0, "Flange Size"=0, "Height"=0, "Load Decision"=0, "Cart Insert"=0}}  # Task Details
        # "New serial has arrived at the scanner stage\nand it's valid s.no with existance in DB"
        # "The new serial task is stored in the Functional global\nuntil the robot becomes available. This will help unwanted \nqueueing of serial tasks in ROBO FIFO queue, when the operator\nis removing/replacing the motor.\nStation to Load will be determined\nin the Robot Controller loop."
        n208 = Unbundle By Name(w521) -> ("Serial No"=w520:string)
        n209 = call "ALTS-2015 DB Serial Details Driver.vi"("Serial Number"=w520, "Operation"=ALTS-2015_DB_Driver_Options."Read DB", "error in (no error)"=w524) -> ("Serial Details from DB"=w519:T39, "error out"=w523:errorcluster)  [unwired: 10 in, 1 out]
        n210 = Bundle By Name(cluster=w517, "New Serial?"=TRUE ("New Part?"), "Serial No"=w520, "Serial Details"=w519, "Robot Task"=ALTS-2015_Robot_Tasks."Load", "Invalid Serial?"=FALSE) -> (w515:T38)
        n211 = call "ALTS-2015 Serial Task Enqueue Handler FGV.vi"("Command"=ALTS-2015_Serial_Task_Handler_FGV-Command."Set Replace/Insert Falg", "Error In"=w523, "Task Details In"=w515) -> ("Error Out"=w522:errorcluster)  [unwired: 6 in, 2 out]
      }
      frame ">Enqueue Invalid Serial Task" {
        w534 = T38 {"Robot Task"=enum."Load", "Serial No"="", "New Serial?"=FALSE, "Station # Unload"=enum."Station 1", "Last Test Result"=FALSE, "Rerun?"=FALSE, "Station # Rerun"=enum."Station 1", "Invalid Serial?"=FALSE, "Serial Details"={"Adapter Plate Size"=0, "Air Leak Test Type "=0, "Displacement Size"=0, "Flange Size"=0, "Height"=0, "Load Decision"=0, "Cart Insert"=0}}  # Task Details
        # "The new serial task is stored in the Functional global\nuntil the robot becomes available. This will help unwanted \nqueueing of serial tasks in ROBO FIFO queue, when the operator\nis removing/replacing the motor."
        # "Invalid serial task is sent when the serial number scanned is invalid or not present in DB (Load decision will not affect in this case). Robot should move it to bin."
        n212 = Unbundle By Name(w528) -> ("Serial No"=w527:string)
        n213 = Bundle By Name(cluster=w534, "New Serial?"=TRUE ("New Part?"), "Invalid Serial?"=TRUE, "Robot Task"=ALTS-2015_Robot_Tasks."Invalid Serial", "Serial No"=w527) -> (w532:T38)
        n214 = call "ALTS-2015 Serial Task Enqueue Handler FGV.vi"("Command"=ALTS-2015_Serial_Task_Handler_FGV-Command."Set Replace/Insert Falg", "Error In"=w535, "Task Details In"=w532) -> ("Error Out"=w531:errorcluster)  [unwired: 6 in, 2 out]
      }
      frame ">Enqueue Rerun Task" {
        n215 = Unbundle By Name(w543) -> ("Stations to Rerun"=w542:T23[])
        n216 = call "ALTS-2015 Enqueue Rerun Task State.vi"("error in (no error)"=w545, "Stations to Rerun In"=w542) -> ("error out"=w544:errorcluster, "Stations to Rerun Out"=w539:T23[])  [unwired: 8 in]
        n217 = Empty Array?(array=w539) -> (empty?=w540:bool)
        n218 = Bundle By Name(cluster=w543, "Stations to Rerun"=w539) -> (w541:T34)
        n219 = case shown="False" w540 {
          tunnel: w538 -> [w547 w551]
          tunnel: [w546 w551] -> w537
          frame False {
            # "Execute this case again if rerun \ntasks are not enqueued completely."
            n220 = Format Into String(format string="%s%s", initial string=w547, ALTS-2015_Auto_Main_Screen_States.">Poll", ALTS-2015_Auto_Main_Screen_States.">Enqueue Rerun Task" ("input 2")) -> (resulting string=w546:string)  [unwired: 1 in, 1 out]
          }
          frame True {
          }
        }
      }
      frame ">Enqueu Unload Task" {
        n221 = Unbundle By Name(w559) -> ("Unload Task"=w557:T30[])
        n222 = call "ALTS-2015 Enqueue Unload Task State.vi"("error in (no error)"=w560, "Unload Tasks In"=w557) -> ("error out"=w558:errorcluster, "Unload Tasks Out"=w553:T30[])  [unwired: 8 in]
        n223 = Empty Array?(array=w553) -> (empty?=w552:bool)
        n224 = Bundle By Name(cluster=w559, "Unload Task"=w553) -> (w556:T34)
        n225 = case shown="False" w552 {
          tunnel: w555 -> [w562 w566]
          tunnel: [w561 w566] -> w554
          frame False {
            # "Execute this case if unload tasks\nare not enqueued completely."
            n226 = Format Into String(format string="%s%s", initial string=w562, ALTS-2015_Auto_Main_Screen_States.">Poll", ALTS-2015_Auto_Main_Screen_States.">Enqueu Unload Task" ("input 2")) -> (resulting string=w561:string)  [unwired: 1 in, 1 out]
          }
          frame True {
          }
        }
      }
    }
  }
  n227 = while {
    tunnel: [w567] -> w6
    tunnel: w5 -> [w567]
    stop <- w568 stop-if-true
    # "Delay to run  OPC Engine before\nrunning following nodes."
    n228 = Wait (ms)(milliseconds to wait=u32 100) -> ()  [unwired: 1 out]
    n229 = call "ALTS-2015 OPC LV2 Global.vi"("Option"=ALTS-2015_OPC_Global_Options."Read 1", "Elements"=ALTS-2015_OPC_Global_Elements."OPC - W Running") -> ("Status Out"=w574:bool)  [unwired: 7 in, 2 out]
    n230 = call "ALTS-2015 OPC LV2 Global.vi"("Option"=ALTS-2015_OPC_Global_Options."Read 1", "Elements"=ALTS-2015_OPC_Global_Elements."OPC - R Running") -> ("Status Out"=w573:bool)  [unwired: 7 in, 2 out]
    n231 = And(x=w573, y=w574) -> (x .and. y?=w568:bool)
  }
  n232 = while {
    shift-right: [w576] -> w19
    shift-left: w5 -> [w583]
    stop <- w580 stop-if-true
    # "31.01.13\n\nHandled read test data result and write result to DataBase in the loop below to avoid the GUI getting held because of wait time(5 Secs)."
    n233 = call "ALTS-2015 LV2GBL Queue.vi"("Enum"=enum16{"Init", "Enqueue", "Dequeue", "Destroy"}."Dequeue", "error in (no error)"=w583) -> ("error out"=w581:errorcluster, "Dequeued Element"=w579:T24)  [unwired: 8 in]
    n234 = Unbundle By Name(w579) -> ("Test Status"=w578:string, "Station Name"=w577:T23)
    n235 = case shown="\"Fail\", \"Pass\"" w578 {
      selector: w578 -> [_ w590 _]
      tunnel: w581 -> [w585 w591 w628]
      tunnel: [w584 w587 w626] -> w576
      tunnel: [_ _ TRUE] -> w580
      tunnel: w577 -> [_ w589 _]
      frame "", Default {
        n236 = call <vilib>:"Clear Errors.vi"("error in (no error)"=w585) -> ("error out"=w584:errorcluster)  [unwired: 6 in]
      }
      frame "Fail", "Pass" {
        # "Same as Previous Test Result?"
        n237 = case shown="\"Pass\", Default" w590 {
          tunnel: [enum16{"Pass", "Fail"}."Fail" ("Status") enum16{"Pass", "Fail"}."Pass" ("Status")] -> w593
          frame "Fail" {
          }
          frame "Pass", Default {
          }
        }
        n238 = call "ALTS-2015 Read Test Data Result.vi"("error in (no error)"=w591, "Station Enum"=w589, "Status"=w593) -> ("error out"=w598:errorcluster, "Same as Previous Test Result?"=w592:bool)  [unwired: 7 in]
        n239 = call "ALTS-2015 LV2GBL Station Info.vi"("Options"=ALTS-2015_LV2GBL_Station_Info_Options."Read All", "error in"=w598) -> ("error out"=w595:errorcluster, "Station Info Array"=w597:T2[])  [unwired: 7 in, 1 out]
        n240 = To Long Integer(number=w589) -> (32bit integer=w600:i32)
        n241 = Index Array(array=w597, index=w600) -> (element=w596:T2)
        n242 = case shown="\"Station 1\", Default" w589 {
          tunnel: w596 -> [w615 w617 w620 w623]
          tunnel: w595 -> [w614 w618 w621 w624]
          tunnel: [w613 w616 w619 w622] -> w594
          frame "Station 1", Default {
            n243 = property on="Station Cluster" class="Clust (strict)"(error in=w614, "Value"=w615) -> (error out=w613:errorcluster)  [unwired: 1 in, 1 out]
          }
          frame "Station 2" {
            n244 = property on="Station Cluster 2" class="Clust (strict)"(error in=w618, "Value"=w617) -> (error out=w616:errorcluster)  [unwired: 1 in, 1 out]
          }
          frame "Station 3" {
            n245 = property on="Station Cluster 3" class="Clust (strict)"(error in=w621, "Value"=w620) -> (error out=w619:errorcluster)  [unwired: 1 in, 1 out]
          }
          frame "Station 4" {
            n246 = property on="Station Cluster 4" class="Clust (strict)"(error in=w624, "Value"=w623) -> (error out=w622:errorcluster)  [unwired: 1 in, 1 out]
          }
        }
        n247 = case shown="False" w592 {
          tunnel: w594 -> [w605 w612]
          tunnel: [w604 w612] -> w588
          tunnel: w589 -> [w603 _]
          frame False {
            n248 = call "ALTS-2015 Status Message Display.vi"("Status Message Options"=ALTS-2015_Status_Message_Options."Writing Result to DB...", "error in (no error)"=w605, "Station Enum"=w603) -> ("error out"=w610:errorcluster)  [unwired: 7 in, 1 out]
            n249 = call "ALTS-2015 Bundle Cluster for DB Result format.vi"("Options"=ALTS-2015_Bundle_Cluster_for_DB_Result_Options."Write", "error in (no error)"=w610, "Station Enum"=w603) -> ("error out"=w608:errorcluster)  [unwired: 7 in, 1 out]
            n250 = call "ALTS-2015 DB Write Result Driver.vi"("Operation"=ALTS-2015_Write_DB_Write_Result_Driver_Cases."Write Result", "Error In"=w608, "DB Write Result Options"=ALTS-2015_write_DB_Result_cases."Enter All Data") -> ("error out"=w604:errorcluster)  [unwired: 8 in]
          }
          frame True {
          }
        }
        n251 = call "ALTS-2015 LV2GBL Error.vi"("error in - DB Loop"=w588, "Operation"=T5."Set - DB Loop") -> ("error out  - DB Loop"=w587:errorcluster)  [unwired: 8 in, 1 out]
      }
      frame ">Exit" {
        n252 = call "ALTS-2015 LV2GBL Queue.vi"("Enum"=enum16{"Init", "Enqueue", "Dequeue", "Destroy"}."Destroy", "error in (no error)"=w628) -> ("error out"=w626:errorcluster)  [unwired: 8 in, 1 out]
      }
    }
  }
  n253 = call "ALTS-2015 LV2GBL INI Info.vi"("error in"=w5) -> ("error out"=w16:errorcluster, "Configuration Cluster Out"=w15:T35)  [unwired: 9 in]
  n254 = call "ALTS-2015 OPC Engine Main.vi"("error in (no error)"=w5) -> ("error out"=w10:errorcluster)  [unwired: 10 in]
  n255 = Unbundle By Name(w15) -> ("Simulation.Simulate DAQ Hardware"=w14:bool)
  n256 = disable-structure shown="Default" {
    disable-tunnel: w16 -> [w631 w635]
    disable-tunnel: w14 -> [w630 _]
    disable-tunnel: [w629 w635] -> w8
    frame condition #0 (active) {
      n257 = case shown="False" w630 {
        tunnel: [w633 w634] -> w629
        tunnel: w631 -> [w632 w634]
        frame False {
          n258 = call "SLL DE DAQ Engine Main.vi"("error in (no error)"=w632) -> ("error out"=w633:errorcluster)  [unwired: 10 in]
        }
        frame True {
        }
      }
    }
    frame condition #1 {
    }
  }
  n259 = call "Test DAQ OPC and Robot.vi"("error in"=w6) -> ("error out"=w11:errorcluster)  [unwired: 9 in]
  n260 = call "ALTS-2015 Robot Controller Loop.vi"("error in (no error)"=w6) -> ("error out"=w12:errorcluster)  [unwired: 10 in]
  n261 = Merge Errors(w11, w12, w10, w8) -> (w9:errorcluster)
  n262 = Merge Errors(w9, w18, w19) -> (w21:errorcluster)
  n263 = call "ALTS-2015 Close All.vi"("error in"=w21) -> ("error out"=w7:errorcluster)  [unwired: 10 in]
  n264 = call "SLL  Is Exe.vi"("error in (no error)"=w7) -> ("error out"=w2:errorcluster, "Is Exe?"=w3:bool)  [unwired: 9 in]
  n265 = case "App is Exe? Close the GUI" shown="True" w3 {
    tunnel: w2 -> [w636 w638]
    tunnel: [w636 w637] -> w1
    frame False {
    }
    frame True {
      n266 = invoke class="VI" method="FP.Close"(error in=w638) -> (error out=w637:errorcluster)  [unwired: 2 in, 2 out]
    }
  }
  "error out" <- w1
